vi "Interpret Error.vi"(7 "Error In":errorcluster, 11 "Code":i32) -> (0 "Error Out":errorcluster)   [LabVIEW 2018]
uses:
  Instance           1 23Saved   Interpret Error .vi
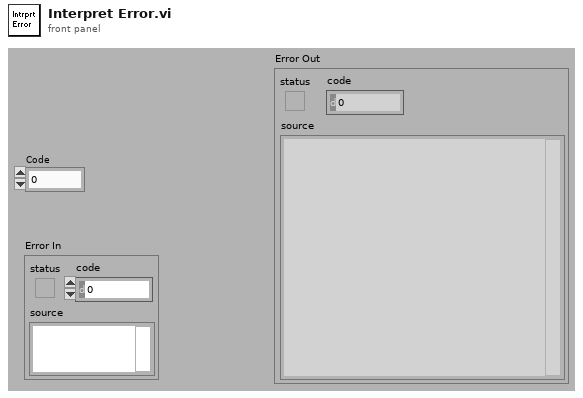
[diagram p1: front panel]
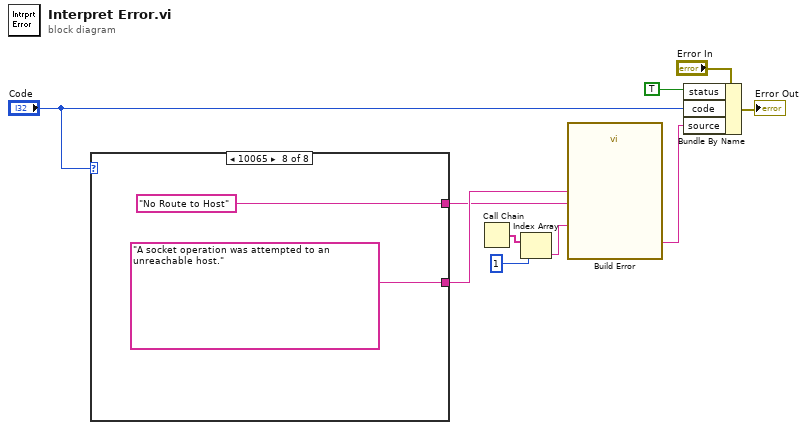
[diagram p0: block diagram]
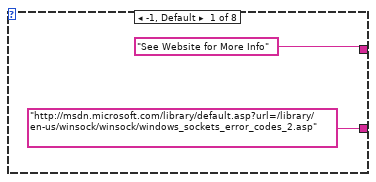
[diagram p2: hidden frame]
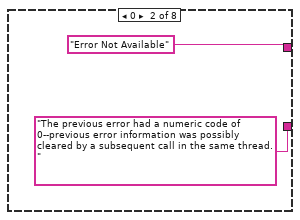
[diagram p3: hidden frame]
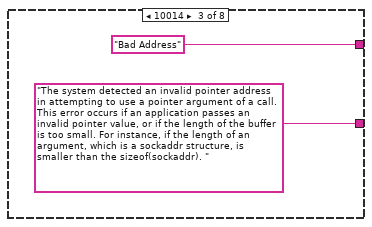
[diagram p4: hidden frame]
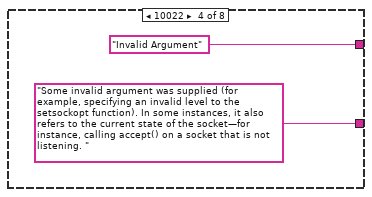
[diagram p5: hidden frame]
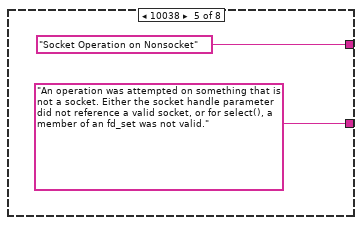
[diagram p6: hidden frame]
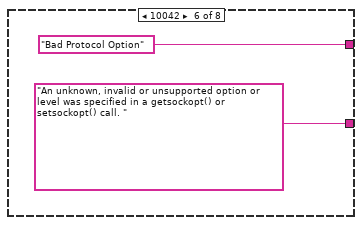
[diagram p7: hidden frame]
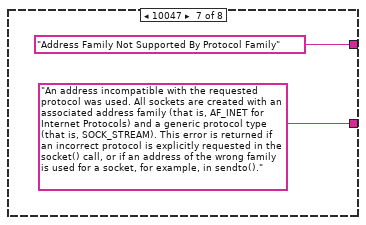
[diagram p8: hidden frame]
diagram:
  n1 = case shown="10065" "Code" {
    tunnel: ["See Website for More Info" "Error Not Available" "Bad Address" "Invalid Argument" "Socket Operation on Nonsocket" "Bad Protocol Option" "Address Family Not Supported By Protocol Family" "No Route to Host"] -> w1
    tunnel: ["http://msdn.microsoft.com/library/default.asp?url=/library/en-us/winsock/winsock/windows_sockets_error_codes_2.asp" "The previous error had a numeric code of 0--previous error information was possibly cleared by a subsequent call in the same thread." "The system detected an invalid pointer address in attempting to use a pointer argument of a call. This error occurs if an application passes an invalid pointer value, or if the length of the buffer is too small. For instance, if the length of an argument, which is a sockaddr structure, is smaller than the sizeof(sockaddr). " "Some invalid argument was supplied (for example, specifying an invalid level to the setsockopt function). In some instances, it also refers to the current state of the socket—for instance, calling accept() on a socket that is not listening. " "An operation was attempted on something that is not a socket. Either the socket handle parameter did not reference a valid socket, or for select(), a member of an fd_set was not valid." "An unknown, invalid or unsupported option or level was specified in a getsockopt() or setsockopt() call. " "An address incompatible with the requested protocol was used. All sockets are created with an associated address family (that is, AF_INET for Internet Protocols) and a generic protocol type (that is, SOCK_STREAM). This error is returned if an incorrect protocol is explicitly requested in the socket() call, or if an address of the wrong family is used for a socket, for example, in sendto()." "A socket operation was attempted to an unreachable host."] -> w3
    frame -1, Default {
    }
    frame 0 {
    }
    frame 10014 {
    }
    frame 10022 {
    }
    frame 10038 {
    }
    frame 10042 {
    }
    frame 10047 {
    }
    frame 10065 {
    }
  }
  n2 = Call Chain() -> (call chain=w4:string[])
  n3 = Index Array(array=w4, index=1) -> (element=w2:string)
  n4 = call "Build Error"("PATH"=w2, "ERROR"=w1, "DESCRIPTION"=w3) -> ("Result"=w7:string)  [unwired: 11 in, 1 out]
  n5 = Bundle By Name(cluster="Error In", "status"=TRUE, "code"="Code", "source"=w7) -> (→"Error Out":errorcluster)
